vi "Line Configuration to Advanced Writer Configuration.vi"(2 "key Name":T1, 3 "Advanced Configuration":T3={"typeName"="", "key Name"=enum."<none>", "domainParticipantQoSProfile"="", "dataWriterQoSProfile"="", "forceArrayMapping?"=FALSE, "forceUnboundedString?"=FALSE, "forceExclusiveReader?"=FALSE, "forceRead? (only ExclusiveReader)"=FALSE, "ContentFilteredTopic Info"={"Filter Type"="DDS_SQLFILTER_NAME", "ContentFilteredTopic Name"="", "Filter Expression"=""}}) -> (1 "Advanced Writer Configuration":T2)   [LabVIEW 2016, in "DDS Custom Device Engine.lvlib"]
uses:
  DDS Custom Device Engine.lvlib
  Shared/Advanced DDS Configuration.ctl
  Shared/key Enum.ctl
  <vilib>/RTI DDS Toolkit/Types/RTI DDS ContentFilteredTopic Info.ctl
  <vilib>/RTI DDS Toolkit/Types/RTI DDS Advanced Writer Configuration.ctl
  <vilib>/RTI DDS Toolkit/Library/LVDDS_library.lvlib
  Shared/DDS Custom Device Shared.lvlib
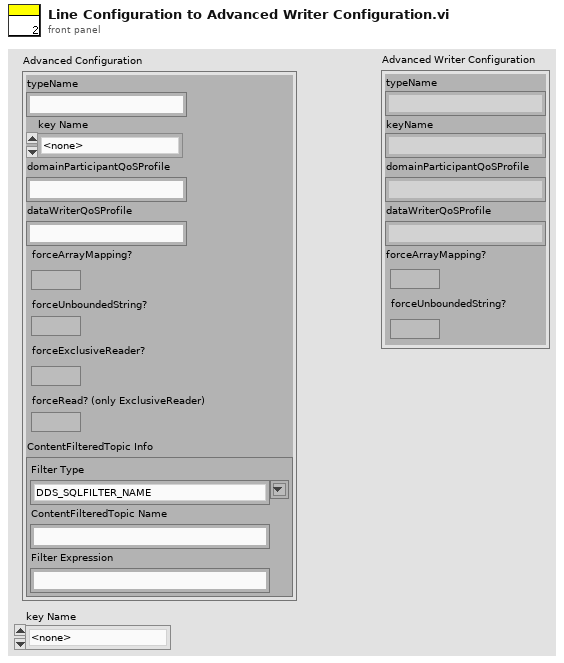
[diagram p1: front panel]
types:
  T1 = typedef "DDS Custom Device Shared.lvlib/key Enum.ctl" = enum16{"<none>", "I32_Num", "I64_Num", "U16_Num", "innercluster.Sgl_Num", "innercluster.Boolean"}
  T2 = typedef "LVDDS_library.lvlib/RTI DDS Advanced Writer Configuration.ctl" = cluster{"typeName":string, "keyName":string, "domainParticipantQoSProfile":string, "dataWriterQoSProfile":string, "forceArrayMapping?":bool, "forceUnboundedString?":bool}
  T3 = typedef "DDS Custom Device Shared.lvlib/Advanced DDS Configuration.ctl" = cluster{"typeName":string, "key Name":T1, "domainParticipantQoSProfile":string, "dataWriterQoSProfile":string, "forceArrayMapping?":bool, "forceUnboundedString?":bool, "forceExclusiveReader?":bool, "forceRead? (only ExclusiveReader)":bool, "ContentFilteredTopic Info":T4}
  T4 = typedef "LVDDS_library.lvlib/RTI DDS ContentFilteredTopic Info.ctl" = cluster{"Filter Type":string, "ContentFilteredTopic Name":string, "Filter Expression":string}
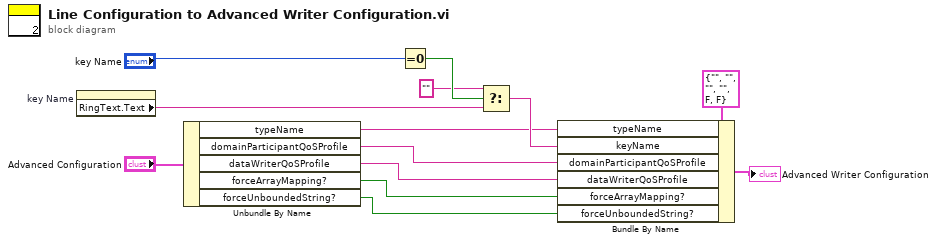
[diagram p0: block diagram]
diagram:
  n1 = property on="key Name" class="Enum (strict)"() -> ("RingText.Text"=w6:string)  [unwired: 2 in, 2 out]
  n2 = Unbundle By Name("Advanced Configuration") -> ("typeName"=w1:string, "domainParticipantQoSProfile"=w3:string, "dataWriterQoSProfile"=w2:string, "forceArrayMapping?"=w10:bool, "forceUnboundedString?"=w9:bool)
  n3 = Equal To 0?(x="key Name") -> (x = 0?=w7:bool)
  n4 = Select(t="", s=w7, f=w6) -> (s? t:f=w4:string)
  n5 = Bundle By Name(cluster=T2 {"typeName"="", "keyName"="", "domainParticipantQoSProfile"="", "dataWriterQoSProfile"="", "forceArrayMapping?"=FALSE, "forceUnboundedString?"=FALSE} ("Advanced Writer Configuration"), "typeName"=w1, "keyName"=w4, "domainParticipantQoSProfile"=w3, "dataWriterQoSProfile"=w2, "forceArrayMapping?"=w10, "forceUnboundedString?"=w9) -> (→"Advanced Writer Configuration":T2)
